vi "Initialize.vi"(8 "error in (no error)":errorcluster, 9 "Marca":string, 10 "Puerto Com":refnum<visa-resource-name>, 11 "object in":refnum<class "Serial Device.lvclass">) -> (0 "error out":errorcluster, 3 "object out":refnum<class "Serial Device.lvclass">)   [LabVIEW 2020, in "Serial Device.lvclass"]
uses:
  Serial Device.lvclass
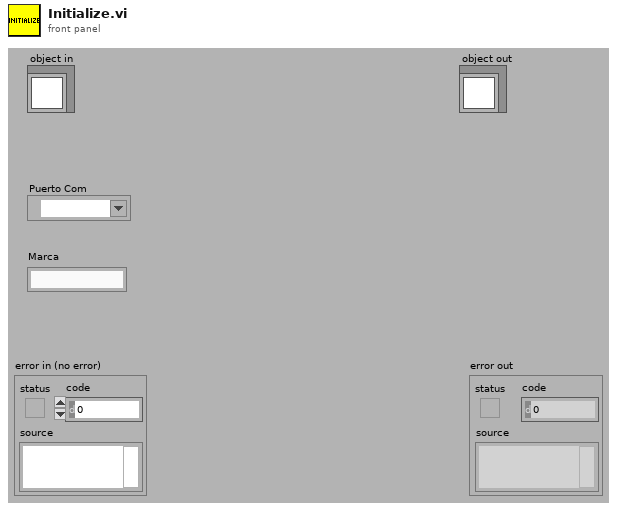
[diagram p1: front panel]
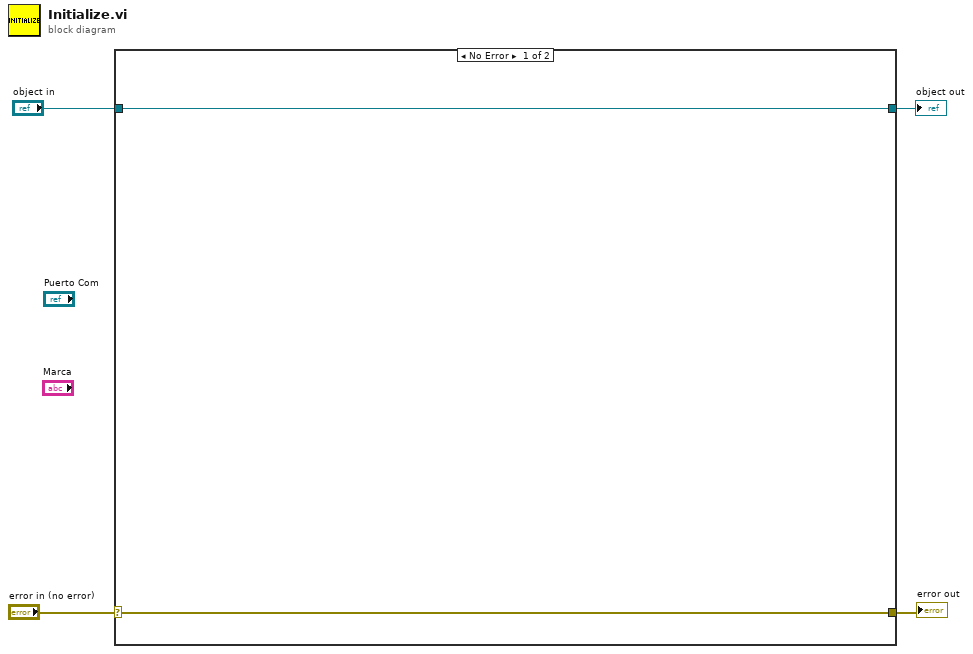
[diagram p0: block diagram]
diagram:
  n1 = case shown="No Error" "error in (no error)" {
    selector: "error in (no error)" -> [w6 w8]
    tunnel: [w6 w8] -> w3
    tunnel: [w5 w7] -> w1
    tunnel: "object in" -> [w5 w7]
    frame No Error {
    }
    frame Error {
    }
  }
  "error out" <- w3
  "object out" <- w1
